vi "DSF.Engine.Transceiver.Initialize.vi"(8 "error in (no error)":errorcluster, 9 "transceiver settings":T1, 10 "Transfer Groups Configurations":refnum<class "DSF.Shared.Configuration.Transfer Group.lvclass">[](array[class]), 11 "Transceiver in":refnum<class "DSF.Transceiver.GE Reflective Memory.lvclass">) -> (0 "error out":errorcluster, 3 "Transceiver out":refnum<class "DSF.Transceiver.GE Reflective Memory.lvclass">)   [LabVIEW 2017, in "DSF.Transceiver.GE Reflective Memory.lvlib" / "DSF.Transceiver.GE Reflective Memory.lvclass"]
uses:
  DSF.Transceiver.GE Reflective Memory.lvclass
  DSF Core/Built/Engine/DSF.Engine.lvlibp/Shared/Classes/Transfer Group/DSF.Shared.Configuration.Transfer Group.lvclass
  DSF Core/Built/Engine/DSF.Engine.lvlibp/DSF Configuration API/1.0.0/Public/Controls/DSF Settings Info.ctl
  DSF.Transceiver.GE Reflective Memory.lvclass/DSF.Transceiver.GE Reflective Memory.ctl
  <vilib>/NI/GE Reflective Memory Driver/Typedefs/GE 5565PIORC.Typedef.DMA Wait Mode.ctl
  <vilib>/NI/GE Reflective Memory Driver/GE 5565PIORC.lvclass
  DSF Core/Built/Engine/DSF.Engine.lvlibp/DSF Configuration API/1.0.0/DSF Configuration API.lvlib
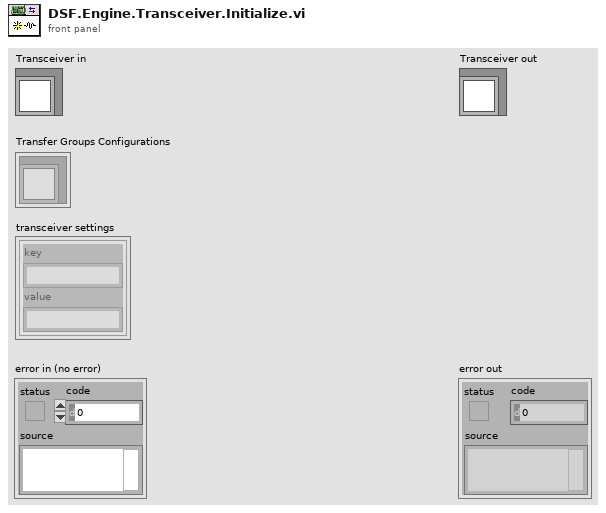
[diagram p1: front panel]
types:
  T1 = typedef "DSF.Engine.lvlibp/DSF Configuration API.lvlib/DSF Settings Info.ctl" = cluster{"key":string, "value":string}[]
  T2 = typedef "GE 5565PIORC.lvclass/GE 5565PIORC.Typedef.DMA Wait Mode.ctl" = enum16{"Polling", "Interrupt"}
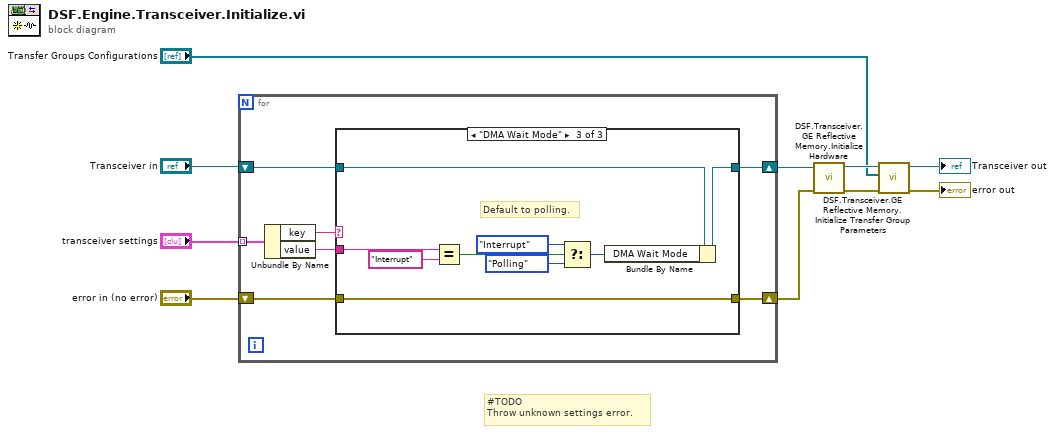
[diagram p0: block diagram]
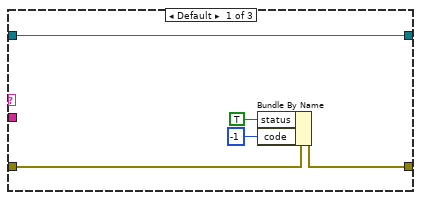
[diagram p2: hidden frame]
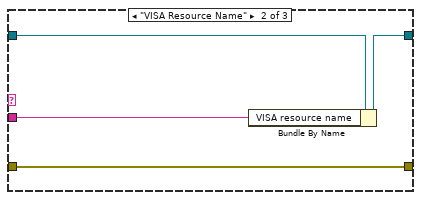
[diagram p3: hidden frame]
diagram:
  # "#TODO\nThrow unknown settings error."
  n1 = for {
    tunnel: "transceiver settings" -> [w17] mode=indexing
    shift-right: [w13] -> w9
    shift-left: "Transceiver in" -> [w14]
    shift-right: [w11] -> w6
    shift-left: "error in (no error)" -> [w12]
    n2 = Unbundle By Name(w17) -> ("key"=w16:string, "value"=w15:string)
    n3 = case shown="\"DMA Wait Mode\"" w16 {
      tunnel: w15 -> [_ w23 w32]
      tunnel: w14 -> [w22 w26 w35]
      tunnel: [w22 w25 w34] -> w13
      tunnel: w12 -> [w21 w24 w33]
      tunnel: [w20 w24 w33] -> w11
      frame Default {
        n4 = Bundle By Name(cluster=w21, "status"=TRUE, "code"=-1) -> (w20:errorcluster)
      }
      frame "VISA Resource Name" {
        n5 = Bundle By Name(cluster=w26, "VISA resource name"=w23) -> (w25:refnum<class "DSF.Transceiver.GE Reflective Memory.lvclass">)
      }
      frame "DMA Wait Mode" {
        # "Default to polling."
        n6 = Equal?(x=w32, y="Interrupt") -> (x = y?=w30:bool)
        n7 = Select(t=GE_5565PIORC.Typedef.DMA_Wait_Mode."Interrupt" ("DMA Wait Mode"), s=w30, f=GE_5565PIORC.Typedef.DMA_Wait_Mode."Polling" ("DMA Wait Mode")) -> (s? t:f=w29:T2)
        n8 = Bundle By Name(cluster=w35, "DMA Wait Mode"=w29) -> (w34:refnum<class "DSF.Transceiver.GE Reflective Memory.lvclass">)
      }
    }
  }
  n9 = call "DSF.Transceiver.GE Reflective Memory.Initialize Hardware.vi"("error in (no error)"=w6, "DSF GE Reflective Memory Transceiver in"=w9) -> ("error out"=w4:errorcluster, "DSF GE Reflective Memory Transceiver out"=w5:refnum<class "DSF.Transceiver.GE Reflective Memory.lvclass">)  [unwired: 8 in]
  n10 = call "DSF.Transceiver.GE Reflective Memory.Initialize Transfer Group Parameters.vi"("error in (no error)"=w4, "Transfer Groups Configurations"="Transfer Groups Configurations", "DSF GE Reflective Memory Transceiver in"=w5) -> ("error out"=→"error out":errorcluster, "DSF GE Reflective Memory Transceiver out"=→"Transceiver out":refnum<class "DSF.Transceiver.GE Reflective Memory.lvclass">)  [unwired: 7 in]
